vi "Acknowledge Shutdown.vi"(8 "error in (no error)":errorcluster, 11 "Plugin Thread in":refnum<class "Plugin Thread.lvclass">) -> (0 "error out":errorcluster, 3 "Plugin Thread out":refnum<class "Plugin Thread.lvclass">)   [LabVIEW 2020, in "DSF Core.lvlib" / "Plugin Thread.lvclass"]
uses:
  Plugin Thread.lvclass
  Interface/Plugin/Response.ctl
  Interface/Plugin/Plugin Interface.lvclass
  Interface/Plugin/Response Parameters.ctl
  Interface/Plugin/Response Data.ctl
  Thread.lvclass
  C:/Users/nitest/Desktop/Git/niveristand-data-sharing-framework-custom-device/Source/Core/Classes/Thread/Thread.lvclass
  C:/Users/nitest/Desktop/Git/niveristand-data-sharing-framework-custom-device/Source/Core/Classes/Thread/Plugin/Plugin Thread.lvclass
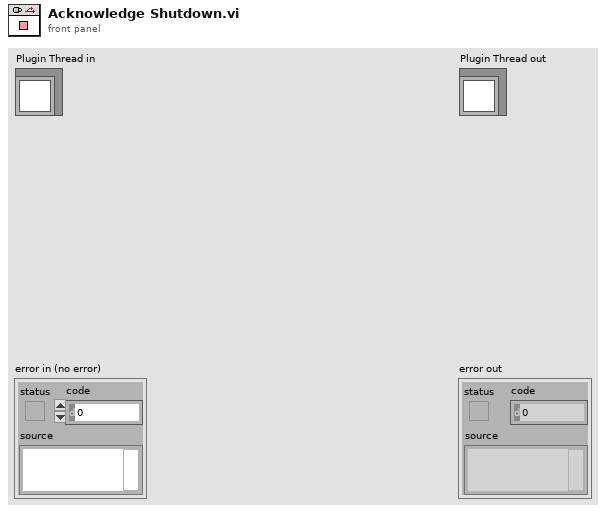
[diagram p1: front panel]
types:
  T1 = typedef "DSF Core.lvlib/Plugin Interface.lvclass/Response Data.ctl" = cluster{"Response":T2, "Parameters":T3}
  T2 = typedef "DSF Core.lvlib/Plugin Interface.lvclass/Response.ctl" = enum8{"General Ack", "Shutting Down"}
  T3 = typedef "DSF Core.lvlib/Plugin Interface.lvclass/Response Parameters.ctl" = cluster{"arg1":u64, "arg2":u64}
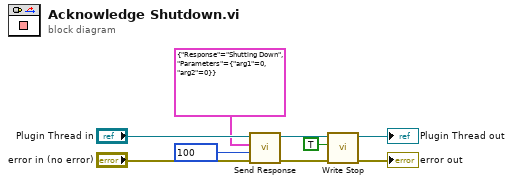
[diagram p0: block diagram]
diagram:
  n1 = call "Send Response.vi"("error in (no error)"="error in (no error)", "timeout in ms (0)"=100, "response"=T1 {"Response"=enum."Shutting Down", "Parameters"={"arg1"=0, "arg2"=0}}, "Plugin Thread in"="Plugin Thread in") -> ("error out"=w4:errorcluster, "Plugin Thread out"=w5:refnum<class "Plugin Thread.lvclass">)  [unwired: 6 in]
  n2 = call "Write Stop.vi"("error in (no error)"=w4, "stop"=TRUE, "Thread in"=w5) -> ("error out"=→"error out":errorcluster, "Thread out"=→"Plugin Thread out":refnum<class "Plugin Thread.lvclass">)  [unwired: 7 in]
